vi "Extract_Igor_TOF_v4.vi"(0 "Master Staging List":T2[](array[typedef]) {"Ramp Step" min=0.0 format="%#_6p"}, 1 "Master AO Table":string[][](table), 2 "Imaging resonance":dbl, 3 "error in (no error)":errorcluster, 4 "Current Variable settings":T1[](array[typedef])) -> (5 "Igor Instruction String":string[](array[string]), 6 "error out":errorcluster)   [LabVIEW 2012]
doc: "This VI extracts the TOF marker information from a stageing list."
uses:
  StagingListEntry.ctt
  StagingListMarkers.ctt
  StagingListOptions.ctt
  TypeDefs/Active procedure variables.ctl
  SubVIs.lvlib
  Controls.llb/Controls.lvlib
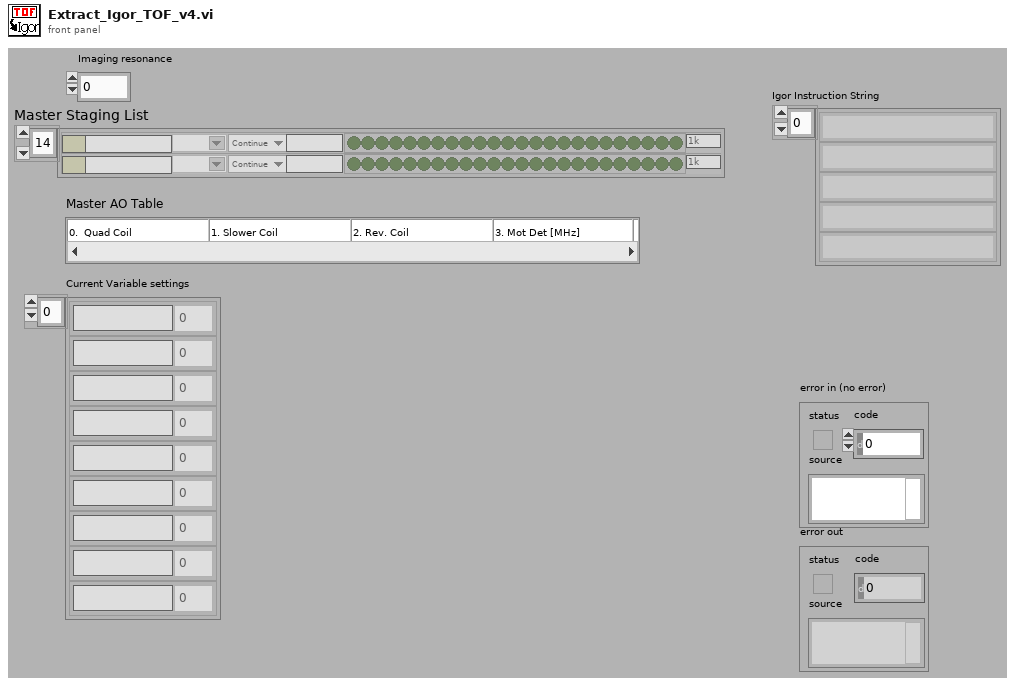
[diagram p1: front panel]
types:
  T1 = typedef "Active procedure variables.ctl" = cluster{"Procedure variable":string, "Value":dbl}
  T2 = typedef "Controls.lvlib/StagingListEntry.ctt" = cluster{"Marker":T3, "Mode":T4, "Output Bits":bool[], "Delay (s)":string, "Ramp Step":dbl, "String":string, "Line Number":string}
  T3 = typedef "Controls.lvlib/StagingListMarkers.ctt" = string
  T4 = typedef "Controls.lvlib/StagingListOptions.ctt" = enum16{"Continue", "Ramp", "Loop", "EndLoop", "Halt"}
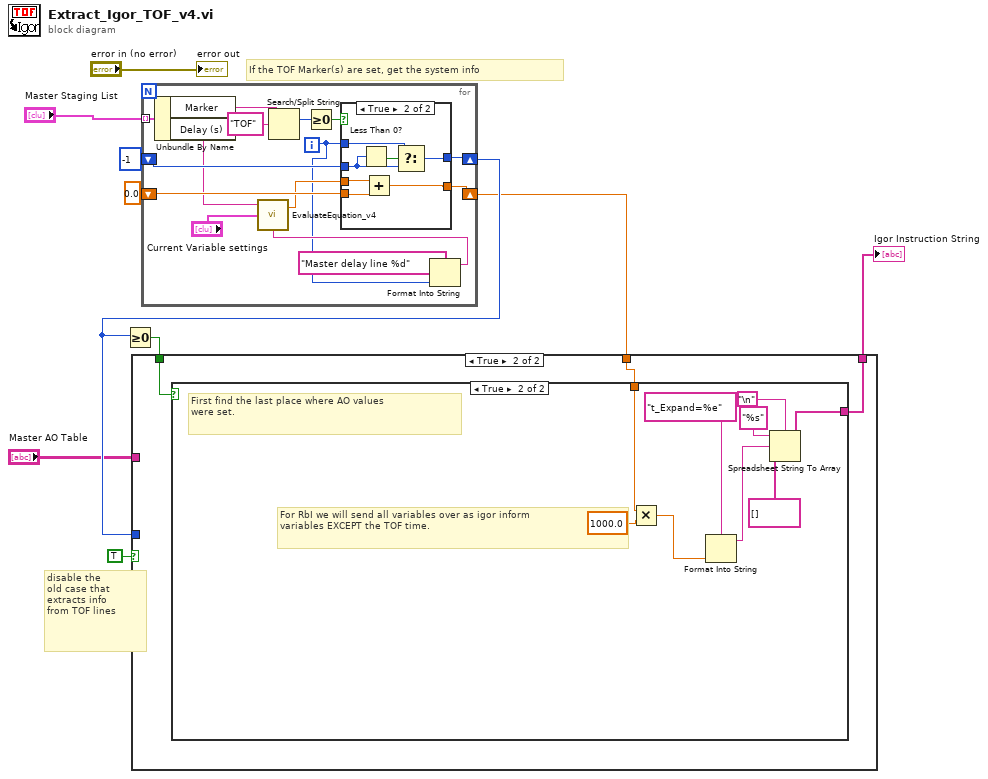
[diagram p0: block diagram]
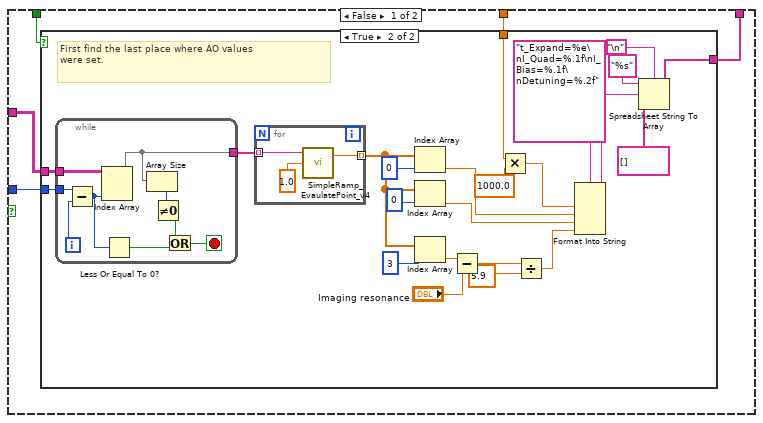
[diagram p2: hidden frame]
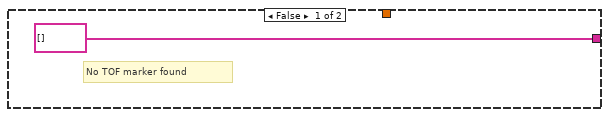
[diagram p3: hidden frame]
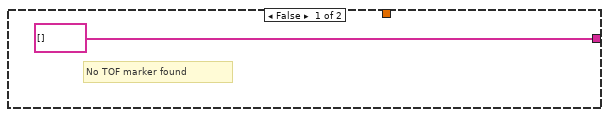
[diagram p4: hidden frame]
diagram:
  # "disable the\nold case that\nextracts info\nfrom TOF lines"
  # "If the TOF Marker(s) are set, get the system info"
  n1 = for {
    tunnel: "Master Staging List" -> [w25] mode=indexing
    shift-right: [w19] -> w7
    shift-left: 0.0 -> [w20]
    shift-right: [w17] -> w9
    shift-left: -1 -> [w18]
    i -> [w11]
    n2 = Unbundle By Name(w25) -> ("Marker"=w23:T3, "Delay (s)"=w15:string)
    n3 = Search/Split String(string=w23, search string/char (-)="TOF") -> (offset of match=w22:i32)  [unwired: 3 out]
    n4 = Greater Or Equal To 0?(x=w22) -> (x >= 0?=w21:bool)
    n5 = Format Into String(format string="Master delay line %d", w11) -> (resulting string=w12:string)  [unwired: 2 in, 1 out]
    n6 = call "EvaluateEquation_v4.vi"("Error Locator"=w12, "Current Variable settings"="Current Variable settings", "formula"=w15) -> ("y value"=w14:dbl)  [unwired: 1 in, 1 out]
    n7 = case shown="True" w21 {
      tunnel: w20 -> [w27 w33]
      tunnel: [w27 w32] -> w19
      tunnel: w14 -> [_ w34]
      tunnel: w18 -> [w26 w30]
      tunnel: w11 -> [_ w29]
      tunnel: [w26 w31] -> w17
      frame False {
      }
      frame True {
        n8 = Less Than 0?(x=w30) -> (x < 0?=w28:bool)
        n9 = Add(x=w34, y=w33) -> (x+y=w32:dbl)
        n10 = Select(t=w29, s=w28, f=w30) -> (s? t:f=w31:i32)
      }
    }
  }
  n11 = Greater Or Equal To 0?(x=w9) -> (x >= 0?=w5:bool)
  n12 = case shown="True" TRUE {
    tunnel: w9 -> [w39 _]
    tunnel: w7 -> [w38 w78]
    tunnel: w5 -> [w37 w76]
    tunnel: [w36 w77] -> w3
    tunnel: "Master AO Table" -> [w35 _]
    frame False {
      n13 = case shown="True" w37 {
        tunnel: [string[] [] w59] -> w36
        tunnel: w35 -> [_ w44]
        tunnel: w38 -> [_ w52]
        tunnel: w39 -> [_ w45]
        frame False {
          # "No TOF marker found"
        }
        frame True {
          # "First find the last place where AO values \nwere set."
          n14 = while {
            tunnel: w45 -> [w75]
            tunnel: w44 -> [w73]
            tunnel: [w67] -> w42
            i -> [w74]
            stop <- w71 stop-if-true
            n15 = Subtract(x=w75, y=w74) -> (x-y=w72:i32)
            n16 = Index Array(array=w73, index (row)=w72) -> (element=w67:string[])  [unwired: 1 in]
            n17 = Less Or Equal To 0?(x=w72) -> (x <= 0?=w70:bool)
            n18 = Array Size(array=w67) -> (size(s)=w68:i32)
            n19 = Not Equal To 0?(x=w68) -> (x != 0?=w69:bool)
            n20 = Or(x=w69, y=w70) -> (x .or. y?=w71:bool)
          }
          n21 = for {
            tunnel: w42 -> [w66] mode=indexing
            tunnel: [w65] -> w41 mode=indexing
            n22 = call "SimpleRamp_EvaulatePoint_v4.vi"("Time"=1.0, "formula"=w66) -> ("y value"=w65:dbl)  [unwired: 1 in, 1 out]
          }
          n23 = Index Array(array=w41, index=0) -> (element=w56:dbl)
          n24 = Index Array(array=w41, index=0) -> (element=w54:dbl)
          n25 = Index Array(array=w41, index=3) -> (element=w49:dbl)
          n26 = Subtract(x=w49, y="Imaging resonance") -> (x-y=w48:dbl)
          n27 = Multiply(x=w52, y=1000.0) -> (x*y=w51:dbl)
          n28 = Divide(x=w48, y=5.9) -> (x/y=w46:dbl)
          n29 = Format Into String(format string="t_Expand=%e\nI_Quad=%.1f\nI_Bias=%.1f\nDetuning=%.2f", w51, w56, w54, w46) -> (resulting string=w60:string)  [unwired: 2 in, 1 out]
          n30 = Spreadsheet String To Array(delimiter (Tab)="\n", format string="%s", spreadsheet string=w60, array type (2D Dbl)=string[] []) -> (array=w59:string[])
        }
      }
    }
    frame True {
      n31 = case shown="True" w76 {
        tunnel: [string[] [] w84] -> w77
        tunnel: w78 -> [_ w82]
        frame False {
          # "No TOF marker found"
        }
        frame True {
          # "For RbI we will send all variables over as igor inform\nvariables EXCEPT the TOF time."
          # "First find the last place where AO values \nwere set."
          n32 = Multiply(x=w82, y=1000.0) -> (x*y=w81:dbl)
          n33 = Format Into String(format string="t_Expand=%e", w81) -> (resulting string=w85:string)  [unwired: 2 in, 1 out]
          n34 = Spreadsheet String To Array(delimiter (Tab)="\n", format string="%s", spreadsheet string=w85, array type (2D Dbl)=string[] []) -> (array=w84:string[])
        }
      }
    }
  }
  "Igor Instruction String" <- w3
  "error out" <- "error in (no error)"
